vi "Get Number of Scripts.vi"(8 "error in (no error)":errorcluster, 11 "Schedule in":refnum<class "Schedule.lvclass">) -> (0 "error out":errorcluster, 2 "No. of Scripts":u32, 3 "Schedule out":refnum<class "Schedule.lvclass">)   [LabVIEW 2020, in "TALOS.lvlib" / "Run Utilities.lvlib" / "Schedule.lvclass"]
doc: "Get number of all Run instances in the schedule (sum of all the repetitions in the cells)"
uses:
  Schedule.lvclass
  Schedule.lvclass/Schedule.ctl
  Cell/Schedule Cell.lvclass
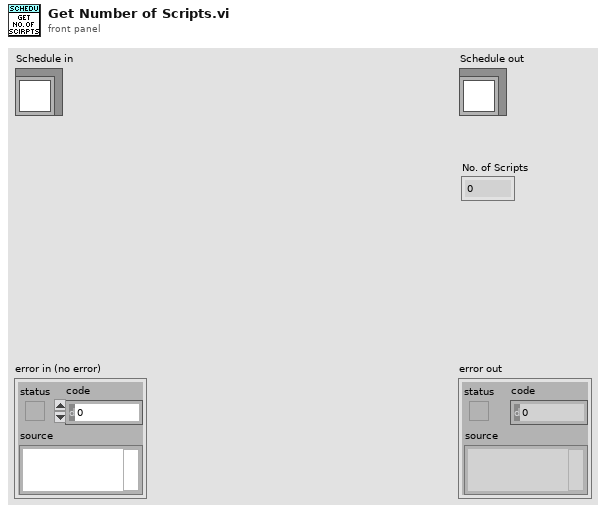
[diagram p1: front panel]
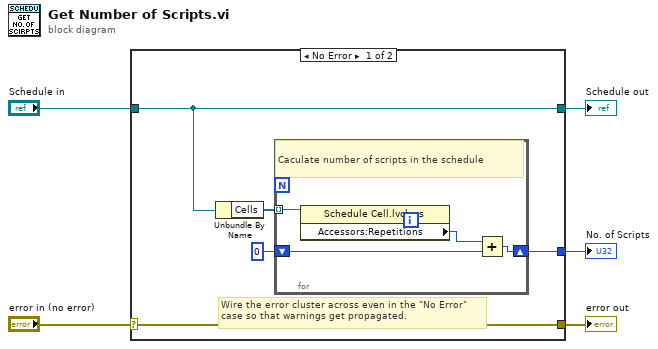
[diagram p0: block diagram]
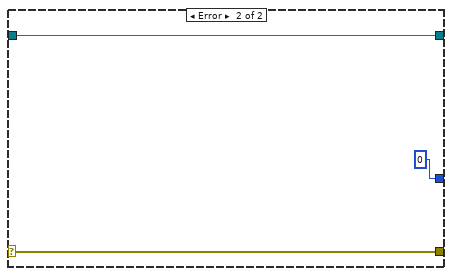
[diagram p2: hidden frame]
diagram:
  n1 = case shown="No Error" "error in (no error)" {
    selector: "error in (no error)" -> [w10 w17]
    tunnel: [w10 w17] -> w4
    tunnel: [w9 w16] -> w2
    tunnel: "Schedule in" -> [w9 w16]
    tunnel: [w6 u32 0 ("y")] -> w1
    frame No Error {
      # "Wire the error cluster across even in the \"No Error\"\ncase so that warnings get propagated."
      n2 = Unbundle By Name(w9) -> ("Cells"=w7:refnum<class "Schedule Cell.lvclass">[])
      n3 = for {
        tunnel: w7 -> [w12] mode=indexing
        shift-right: [w13] -> w6
        shift-left: u32 0 ("y") -> [w14]
        # "Caculate number of scripts in the schedule"
        n4 = property class="Schedule Cell.lvclass"(reference=w12) -> ("Accessors:Repetitions"=w11:u32)  [unwired: 1 in, 2 out]
        n5 = Add(x=w11, y=w14) -> (x+y=w13:u32)
      }
    }
    frame Error {
    }
  }
  "error out" <- w4
  "Schedule out" <- w2
  "No. of Scripts" <- w1
